vi "FTW-STR-Decode-Hex.vi"(7 "Input":string, 11 "error in":errorcluster) -> (8 "Output":string, 15 "error out":errorcluster)   [LabVIEW 2015]
panel:
  # "Inputs"
  # "Outputs"
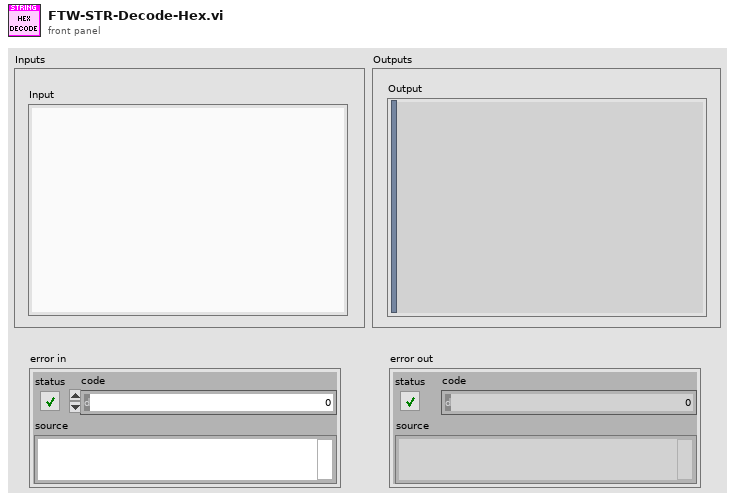
[diagram p1: front panel]
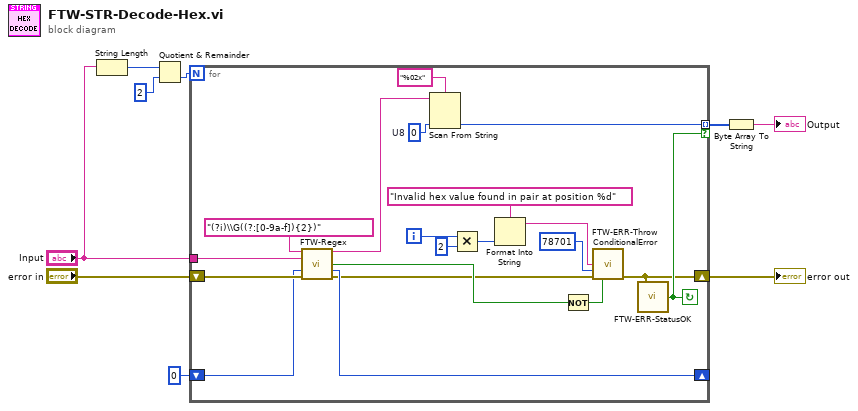
[diagram p0: block diagram]
diagram:
  n1 = String Length(string="Input") -> (length=w6:i32)
  n2 = Quotient & Remainder(x=w6, y=2) -> (floor(x/y)=w4:i32)  [unwired: 1 out]
  n3 = for {
    N: w4 -> [_]
    tunnel: [w27] -> w7 mode=indexing if=w26
    shift-right: [w24] -> w2
    shift-left: "error in" -> [w25]
    shift-right: [w14] -> _
    shift-left: 0 ("Offset after Match") -> [w13]
    tunnel: "Input" -> [w17]
    i -> [w22]
    stop <- w26 continue-if-true
    w28 = u8 0  # U8
    n4 = call "FTW-Regex.vi"("Regular Expression"="(?i)\\G((?:[0-9a-f]){2})", "Input String"=w17, "Starting Offset"=w13, "error in"=w25) -> ("Match"=w15:string, "Match Found?"=w12:bool, "Offset after Match"=w14:i32, "error out"=w10:errorcluster)  [unwired: 7 in, 1 out]
    n5 = Scan From String(format string="%02x", input string=w15, default 1=w28) -> (output 1=w27:u8)  [unwired: 2 in, 3 out]
    n6 = Multiply(x=w22, y=2) -> (x*y=w20:i32)
    n7 = Format Into String(format string="Invalid hex value found in pair at position %d" ("Error Message"), w20) -> (resulting string=w18:string)  [unwired: 2 in, 1 out]
    n8 = Not(x=w12) -> (.not. x?=w11:bool)
    n9 = call "FTW-ERR-ThrowConditionalError.vi"("Error Message"=w18, "Error Code"=78701, "error in"=w10, "Throw Error?"=w11) -> ("error out"=w24:errorcluster)  [unwired: 11 in]
    n10 = call "FTW-ERR-StatusOK.vi"("error to check"=w24) -> ("Status OK?"=w26:bool)
  }
  "error out" <- w2
  n11 = Byte Array To String(unsigned byte array=w7) -> (string=→"Output":string)
